vi "Sub_LinearEquationCoeffCalc.vi"(2 "Lower bound":dbl, 3 "Upper bound":dbl) -> (0 "B":dbl, 1 "A":dbl)   [LabVIEW 2021]
panel:
  # "Inputs:"
  # "Outputs::"
  # "Required:"
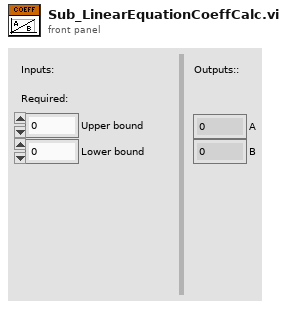
[diagram p1: front panel]
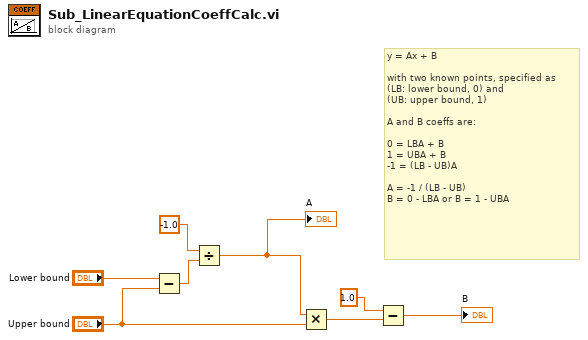
[diagram p0: block diagram]
diagram:
  # "y = Ax + B\n\nwith two known points, specified as \n(LB: lower bound, 0) and \n(UB: upper bound, 1)\n\nA and B coeffs are:\n\n0 = LBA + B\n1 = UBA + B\n-1 = (LB - UB)A\n\nA = -1 / (LB - UB)\nB = 0 - LBA or B = 1 - UBA"
  n1 = Subtract(x="Lower bound", y="Upper bound") -> (x-y=w8:dbl)
  n2 = Divide(x=-1.0, y=w8) -> (x/y=w3:dbl)
  "A" <- w3
  n3 = Multiply(x=w3, y="Upper bound") -> (x*y=w4:dbl)
  n4 = Subtract(x=1.0, y=w4) -> (x-y=→"B":dbl)
